vi "Init Loop Data.vi"(8 "error in (no error)":errorcluster, 11 "AsyncClassTemplate in":refnum<class "AsyncClassTemplate.lvclass">) -> (0 "error out":errorcluster, 3 "Loop Data":T1)   [LabVIEW 2020, in "Vecto.lvlib" / "AsyncClassTemplate.lvclass"]
uses:
  AsyncClassTemplate.lvclass
  Loop Data.ctl
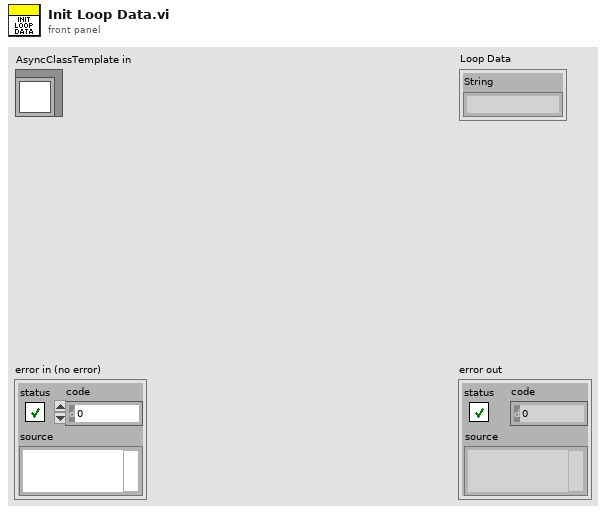
[diagram p1: front panel]
types:
  T1 = typedef "Vecto.lvlib/AsyncClassTemplate.lvclass/Loop Data.ctl" = cluster{"String":string}
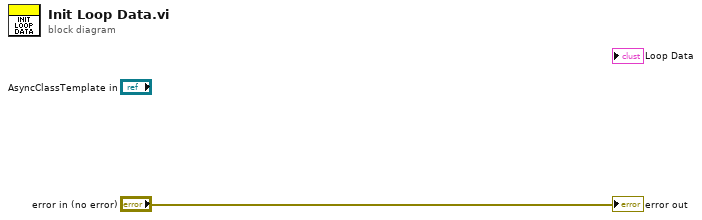
[diagram p0: block diagram]
diagram:
  "error out" <- "error in (no error)"
